vi "Root Folder.vi"() -> (7 "Prefs Root":path)   [LabVIEW 2020, in "User Prefs.lvlib" / "PrefsDB.lvclass"]
uses:
  PrefsDB.lvclass
  <vilib>/Utility/sysdir.llb/System Directory Type.ctl
  PrefsDB.lvclass/PrefsDB.ctl
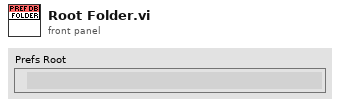
[diagram p1: front panel]
types:
  T1 = typedef "System Directory Type.ctl" = i32
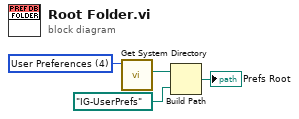
[diagram p0: block diagram]
diagram:
  w4 = T1 4 items=["User Home"=0, "User Desktop"=1, "User Documents"=2, "User Application Data"=3, "User Preferences"=4, "User Temporary"=5, "Public Documents"=6, "Public Application Data"=7, "Public Preferences"=8, "Public Cache"=13, "System Core Libraries"=9, "System Installed Libraries"=10, "Application Files"=11, "Boot Volume Root"=12] ("system directory type")
  n1 = call <vilib>:"Get System Directory.vi"("system directory type"=w4) -> ("system directory"=w3:path)  [unwired: 10 in]
  n2 = Build Path(base path=w3, name or relative path=path "IG-UserPrefs") -> (appended path=→"Prefs Root":path)
